vi "VS-Read Heart Rate (general).vi"(8 "error in (no error)":errorcluster, 11 "Scale":T1={"Slope"=0.0, "Offset"=0.0, "Limits"={"Min"=0.0, "Max"=0.0}, "term config"=-1} {"term config" items=["default"=-1, "RSE"=10083, "NRSE"=10078, "Differential"=10106, "Pseudodifferential"=12529]}) -> (0 "error out":errorcluster, 3 "Heart Rate (bpm)":dbl)   [LabVIEW 2020]
uses:
  Typedefs/PhysMon-Scale.ctl
  epl-vi-lib/Connection VIs/Type Defs/Input sources.ctl
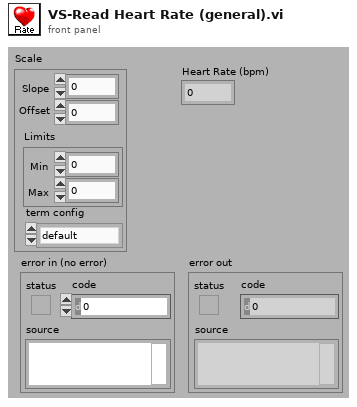
[diagram p1: front panel]
types:
  T1 = typedef "PhysMon-Scale.ctl" = cluster{"Slope":dbl, "Offset":dbl, "Limits":cluster{"Min":dbl, "Max":dbl}, "term config":i32}
  T2 = typedef "Input sources.ctl" = u16
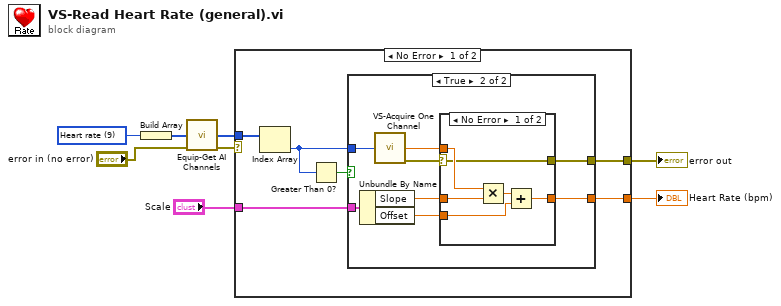
[diagram p0: block diagram]
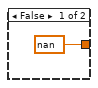
[diagram p2: hidden frame]
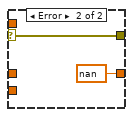
[diagram p3: hidden frame]
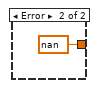
[diagram p4: hidden frame]
diagram:
  w8 = T2 9 items=["--unused--", "Probe Mic Right", "Probe Mic Left", "Cal Mic", "ABR", "CAP Right", "CAP Left", "Startle piezo", "Temperature", "Heart rate"] ("Ring")
  n1 = Build Array(w8) -> (w7:T2[])
  n2 = call "Equip-Get AI Channels.vi"("Inputs"=w7, "error in (no error)"="error in (no error)") -> ("AI Channels"=w6:i32[], "error out"=w5:errorcluster)  [unwired: 12 in]
  n3 = case shown="No Error" w5 {
    tunnel: [w14 nan] -> w4
    tunnel: w6 -> [w13 _]
    tunnel: "Scale" -> [w10 _]
    tunnel: [w9 _] -> w1
    frame No Error {
      n4 = Index Array(array=w13) -> (element=w12:i32)  [unwired: 1 in]
      n5 = Greater Than 0?(x=w12) -> (x > 0?=w11:bool)
      n6 = case shown="True" w11 {
        tunnel: [nan w19] -> w14
        tunnel: w12 -> [_ w22]
        tunnel: w10 -> [_ w21]
        tunnel: [_ w16] -> w9
        frame False {
        }
        frame True {
          n7 = Unbundle By Name(w21) -> ("Slope"=w20:dbl, "Offset"=w18:dbl)
          n8 = call "VS-Acquire One Channel.vi"("index"=w22) -> ("mean"=w23:dbl, "error out"=w17:errorcluster)  [unwired: 13 in]
          n9 = case shown="No Error" w17 {
            selector: w17 -> [w24 w30]
            tunnel: w23 -> [w28 _]
            tunnel: w20 -> [w27 _]
            tunnel: [w26 nan] -> w19
            tunnel: w18 -> [w25 _]
            tunnel: [w24 w30] -> w16
            frame No Error {
              n10 = Multiply(x=w28, y=w27) -> (x*y=w29:dbl)
              n11 = Add(x=w29, y=w25) -> (x+y=w26:dbl)
            }
            frame Error {
            }
          }
        }
      }
    }
    frame Error {
    }
  }
  "error out" <- w1
  "Heart Rate (bpm)" <- w4
